vi "Unpack Message.vi"(8 "error in (no error)":errorcluster, 9 "Packed Message":string, 10 "Message Name":string, 11 "Message Double in":refnum<class "Message Double.lvclass">) -> (0 "error out":errorcluster, 2 "Valid":bool, 3 "Message Double out":refnum<class "Message Double.lvclass">)   [LabVIEW 2016, in "Stream Mediator.lvlib" / "Message Double.lvclass"]
uses:
  <userlib>/Composed Systems/Stream/Mediator/Classes/Message Double/Message Double.lvclass
  C:/Program Files (x86)/National Instruments/LabVIEW 2016/user.lib/Composed Systems/Stream/Mediator/Classes/Message Interface/Message Interface.lvclass
  <userlib>/Composed Systems/Stream/Mediator/Classes/Message Double/Message Double.lvclass/Message Double.ctl
  <vilib>/addons/_JKI.lib/Serialization/JSON/JKI JSON Serialization.lvlib
  <userlib>/Composed Systems/Stream/Mediator/Classes/Message Interface/Message Interface.lvclass
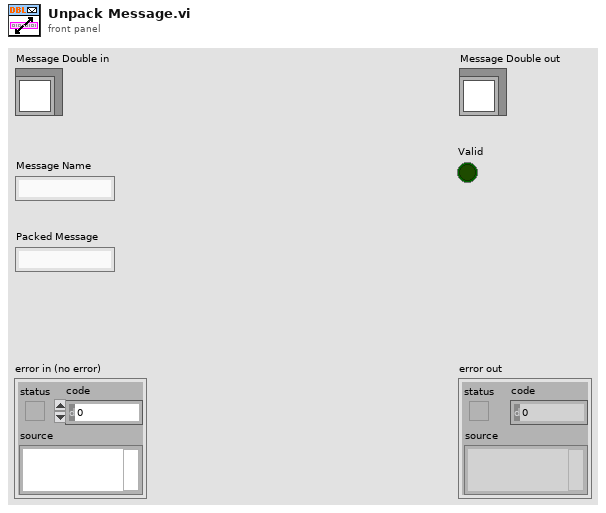
[diagram p1: front panel]
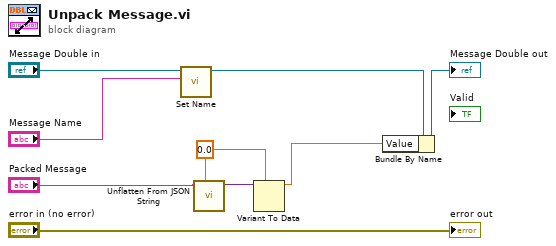
[diagram p0: block diagram]
diagram:
  w4 = 0.0
  n1 = call <userlib>:"Set Name.vi"("Name"="Message Name", "Message Interface in"="Message Double in") -> ("Message Interface out"=w7:refnum<class "Message Double.lvclass">)  [unwired: 8 in, 1 out]
  n2 = call <vilib>:"Unflatten From JSON String.vi"("Type and Defaults"=w4, "JSON String"="Packed Message") -> ("Variant"=w5:variant)  [unwired: 8 in, 1 out]
  n3 = Variant To Data(type=w4, Variant=w5) -> (data=w2:dbl)  [unwired: 1 in, 1 out]
  n4 = Bundle By Name(cluster=w7, "Value"=w2) -> (→"Message Double out":refnum<class "Message Double.lvclass">)
  "error out" <- "error in (no error)"
